vi "HEWH Check Voltage Type.vi"(8 "error in (no error)":errorcluster, 11 "Voltage Array Input":dbl[](array[numeric])) -> (0 "error out":errorcluster, 1 "Voltage_Heating":bool, 2 "Voltage_Min":dbl, 3 "Voltage_Max":dbl)   [LabVIEW 2023]
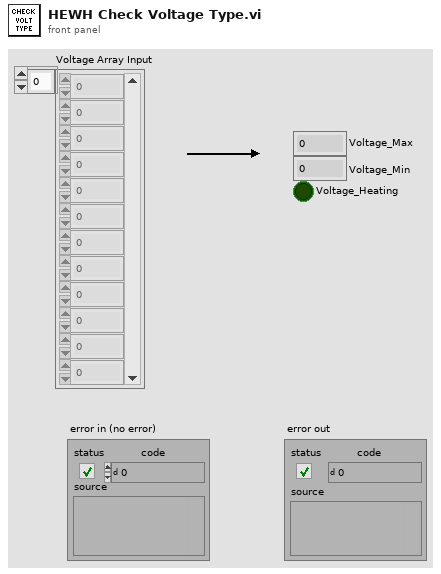
[diagram p1: front panel]
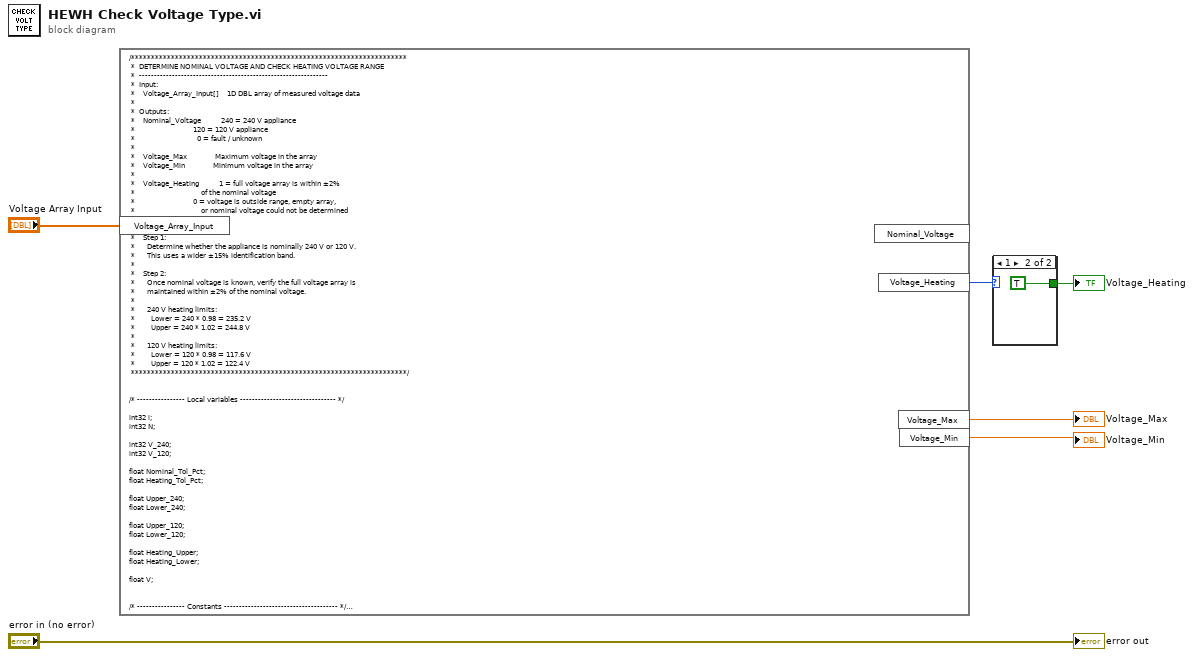
[diagram p0: block diagram]
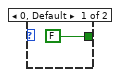
[diagram p2: hidden frame]
diagram:
  n1 = formula code="/*********************************************************************\n *  DETERMINE NOMINAL VOLTAGE AND CHECK HEATING VOLTAGE RANGE\n *  ---------------------------------------------------------------\n *  Input:\n *    Voltage_Array_Input[]    1D DBL array of measured voltage data\n *\n *  Outputs:\n *    Nominal_Voltage          240 = 240 V appliance\n *                             120 = 120 V appliance\n *                               0 = fault / unknown\n *\n *    Voltage_Max              Maximum voltage in the array\n *    Voltage_Min              Minimum voltage in the array\n *\n *    Voltage_Heating          1 = full voltage array is within ±2%\n *                                 of the nominal voltage\n *                             0 = voltage is outside range, empty array,\n *                                 or nominal voltage could not be determined\n *\n *  Logic:\n *    Step 1:\n *      Determine whether the appliance is nominally 240 V or 120 V.\n *      This uses a wider ±15% identification band.\n *\n *    Step 2:\n *      Once nominal voltage is known, verify the full voltage array is\n *      maintained within ±2% of the nominal voltage.\n *\n *      240 V heating limits:\n *        Lower = 240 * 0.98 = 235.2 V\n *        Upper = 240 * 1.02 = 244.8 V\n *\n *      120 V heating limits:\n *        Lower = 120 * 0.98 = 117.6 V\n *        Upper = 120 * 1.02 = 122.4 V\n *********************************************************************/\n\n\n/* ---------------- Local variables -------------------------------- */\n\nint32 i;\nint32 N;\n\nint32 V_240;\nint32 V_120;\n\nfloat Nominal_Tol_Pct;\nfloat Heating_Tol_Pct;\n\nfloat Upper_240;\nfloat Lower_240;\n\nfloat Upper_120;\nfloat Lower_120;\n\nfloat Heating_Upper;\nfloat Heating_Lower;\n\nfloat V;\n\n\n/* ---------------- Constants -------------------------------------- */\n\nNominal_Tol_Pct = 0.15;     /* ±15% band used to identify voltage type */\nHeating_Tol_Pct = 0.02;     /* ±2% band used during heating check      */\n\n\n/* ---------------- Default outputs -------------------------------- */\n\nint32 Nominal_Voltage = 0.0;\n\nVoltage_Max = 0.0;\nVoltage_Min = 0.0;\n\nint32 Voltage_Heating = 0;  /* 0 = out of tolerance, 1 = within tolerance */\n\n\n/* ---------------- Get array length ------------------------------- */\n\nN = sizeOfDim(Voltage_Array_Input, 0);\n\n\n/* ---------------- Calculate nominal identification limits --------- */\n\nUpper_240 = 240.0 * (1.0 + Nominal_Tol_Pct);\nLower_240 = 240.0 * (1.0 - Nominal_Tol_Pct);\n\nUpper_120 = 120.0 * (1.0 + Nominal_Tol_Pct);\nLower_120 = 120.0 * (1.0 - Nominal_Tol_Pct);\n\n\n/* ---------------- Evaluate voltage data --------------------------- */\n\nif (N > 0)\n{\n    /*\n     * Initialize min and max using the first sample.\n     */\n\n    Voltage_Max = Voltage_Array_Input[0];\n    Voltage_Min = Voltage_Array_Input[0];\n\n\n    /*\n     * Start both nominal-voltage checks as TRUE.\n     * If any sample is outside a nominal range,\n     * set that range check to FALSE.\n     */\n\n    V_240 = 1;\n    V_120 = 1;\n\n\n    for (i = 0; i < N; i++)\n    {\n        V = Voltage_Array_Input[i];\n\n\n        /* Track maximum voltage */\n        if (V > Voltage_Max)\n        {\n            Voltage_Max = V;\n        }\n\n\n        /* Track minimum voltage */\n        if (V < Voltage_Min)\n        {\n            Voltage_Min = V;\n        }\n\n\n        /* Check 240 V nominal range */\n        if (V < Lower_240 || V > Upper_240)\n        {\n            V_240 = 0;\n        }\n\n\n        /* Check 120 V nominal range */\n        if (V < Lower_120 || V > Upper_120)\n        {\n            V_120 = 0;\n        }\n    }\n\n\n    /*\n     * Select final nominal voltage.\n     *\n     * Valid:\n     *   V_240 = 1 and V_120 = 0  --> 240 V\n     *   V_240 = 0 and V_120 = 1  --> 120 V\n     *\n     * Fault:\n     *   V_240 = 1 and V_120 = 1\n     *   V_240 = 0 and V_120 = 0\n     */\n\n    if (V_240 == 1 && V_120 == 0)\n    {\n        Nominal_Voltage = 240.0;\n    }\n    else if (V_240 == 0 && V_120 == 1)\n    {\n        Nominal_Voltage = 120.0;\n    }\n    else\n    {\n        Nominal_Voltage = 0.0;\n    }\n\n\n    /*****************************************************************\n     * Heating voltage check.\n        Use Voltage_Min and Voltage_Max:\n     *\n     *   Voltage_Min >= Lower limit\n     *   Voltage_Max <= Upper limit\n     *\n     * If both are true, the full array is inside the allowed range.\n     *****************************************************************/\n\n    if (Nominal_Voltage > 0.0)\n    {\n        Heating_Upper = Nominal_Voltage * (1.0 + Heating_Tol_Pct);\n        Heating_Lower = Nominal_Voltage * (1.0 - Heating_Tol_Pct);\n\n        if (Voltage_Min >= Heating_Lower && Voltage_Max <= Heating_Upper)\n        {\n            Voltage_Heating = 1;\n        }\n        else\n        {\n            Voltage_Heating = 0;\n        }\n    }\n    else\n    {\n        /*\n         * Nominal voltage could not be determined.\n         * Treat heating voltage check as failed.\n         */\n\n        Voltage_Heating = 0;\n    }\n}\nelse\n{\n    /*\n     * Empty array fault.\n     */\n\n    Nominal_Voltage = 0.0;\n\n    Voltage_Max = 0.0;\n    Voltage_Min = 0.0;\n\n    Voltage_Heating = 0;\n}"("Voltage_Array_Input"="Voltage Array Input") -> ("Voltage_Max"=→"Voltage_Max":dbl, "Voltage_Min"=→"Voltage_Min":dbl, "Voltage_Heating"=w2:i32)  [unwired: 1 out]
  n2 = case shown="1" w2 {
    tunnel: [FALSE TRUE] -> w1
    frame 0, Default {
    }
    frame 1 {
    }
  }
  "Voltage_Heating" <- w1
  "error out" <- "error in (no error)"
